vi "(SubVI) Choose Index Interval From an Array_YCC.vi"(3 "End index":i32, 4 "Start index":i32, 6 "array":dbl[](array[numeric])) -> (1 "Array out":dbl[](array[numeric]))   [LabVIEW 2014]
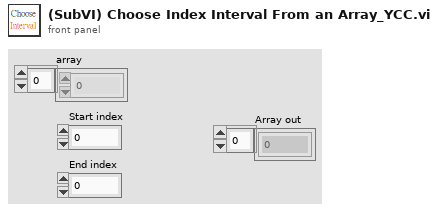
[diagram p1: front panel]
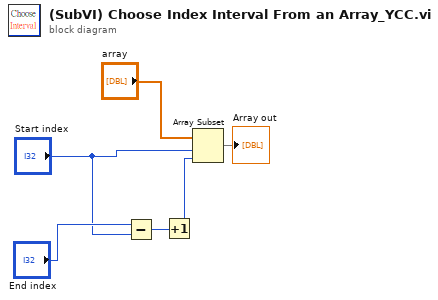
[diagram p0: block diagram]
diagram:
  n1 = Subtract(x="End index", y="Start index") -> (x-y=w3:i32)
  n2 = Increment(x=w3) -> (x+1=w2:i32)
  n3 = Array Subset(array="array", index="Start index", length=w2) -> (→"Array out":dbl[])
